vi "Generate_WF_Class_Dataset.vi"(8 "error in (no error)":errorcluster) -> (0 "error out":errorcluster, 3 "DataSets_All(In1D_Out1D)":T1={"Train"={"Inputs Ref."=variant(refnum<data-value> refnum), "Outputs Ref."=refnum, "Dims_In"=0, "Dataset_Size"=0, "Dims_Out"=0, "Labels"=[], "File Paths"=[]}, "Validation"={"Inputs Ref."=variant(refnum<data-value> refnum), "Outputs Ref."=refnum, "Dims_In"=0, "Dataset_Size"=0, "Dims_Out"=0, "Labels"=[], "File Paths"=[]}, "Test"={"Inputs Ref."=variant(refnum<data-value> refnum), "Outputs Ref."=refnum, "Dims_In"=0, "Dataset_Size"=0, "Dims_Out"=0, "Labels"=[], "File Paths"=[]}})   [LabVIEW 2020]
uses:
  <vilib>/Ngene/Deep Learning Toolkit/Toolkit/NN_Data/API/DataSet/DataSet_Types/NN_DataSets_All(In1D_Out1D).ctl
  <vilib>/Ngene/Deep Learning Toolkit/Toolkit/NN_Data/API/DataSet/DataSet_Types/NN_DataSet(In1D_Out1D).ctl
  <vilib>/Ngene/Deep Learning Toolkit/Toolkit/NN_Data/Controls/DataRef_Types/2D/NN_Data_ref(2D_SGL).ctl
  <vilib>/Ngene/Deep Learning Toolkit/Toolkit/Deep_Learning_Toolkit_by_Ngene.lvlib
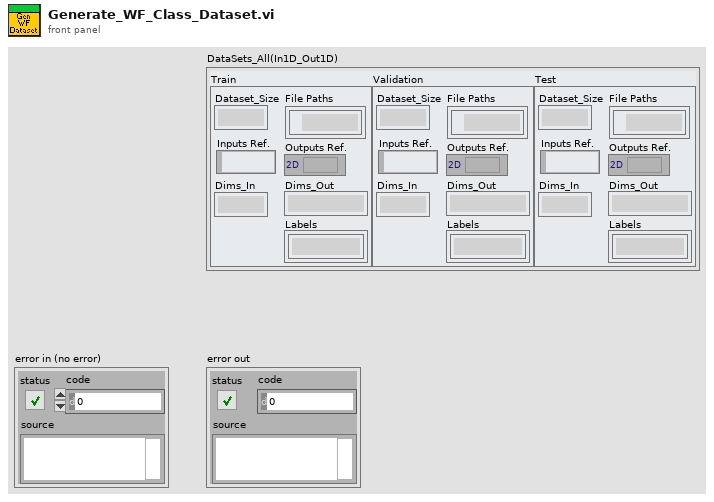
[diagram p1: front panel]
types:
  T1 = typedef "Deep_Learning_Toolkit_by_Ngene.lvlib/NN_DataSets_All(In1D_Out1D).ctl" = cluster{"Train":T2, "Validation":T2, "Test":T2}
  T2 = typedef "Deep_Learning_Toolkit_by_Ngene.lvlib/NN_DataSet(In1D_Out1D).ctl" = cluster{"Inputs Ref.":variant, "Outputs Ref.":T3, "Dims_In":i32, "Dataset_Size":i32, "Dims_Out":i32, "Labels":string[], "File Paths":path[]}
  T3 = typedef "Deep_Learning_Toolkit_by_Ngene.lvlib/NN_Data_ref(2D_SGL).ctl" = refnum<data-value>
  T4 = enum16{"Sine Wave", "Triangle Wave", "Square Wave", "Sawtooth Wave", "Noise"}[]
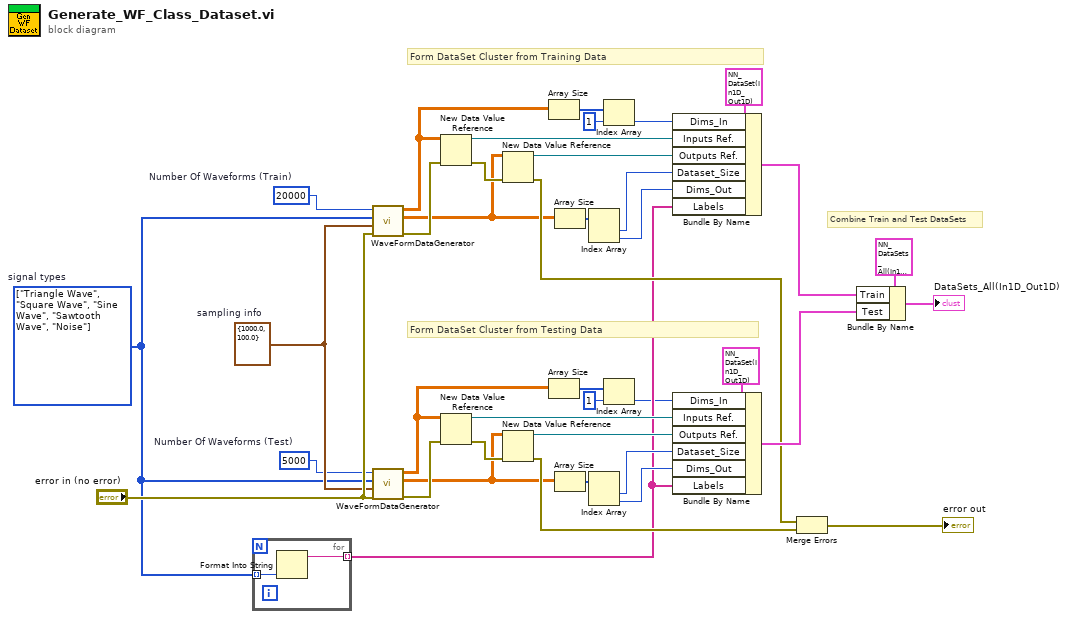
[diagram p0: block diagram]
diagram:
  w31 = 5000  # Number Of Waveforms (Test)
  w37 = cluster{"Fs":dbl, "#s":dbl} {"Fs"=1000.0, "#s"=100.0}  # sampling info
  w12 = 20000  # Number Of Waveforms (Train)
  w5 = T4 [enum."Triangle Wave", enum."Square Wave", enum."Sine Wave", enum."Sawtooth Wave", enum."Noise"] items=["Sine Wave", "Triangle Wave", "Square Wave", "Sawtooth Wave", "Noise"]  # signal types
  # "Combine Train and Test DataSets"
  # "Form DataSet Cluster from Testing Data"
  # "Form DataSet Cluster from Training Data"
  n1 = for {
    tunnel: w5 -> [w41] mode=indexing
    tunnel: [w40] -> w4 mode=indexing
    n2 = Format Into String(w41) -> (resulting string=w40:string)  [unwired: 3 in, 1 out]
  }
  n3 = call "WaveFormDataGenerator.vi"("error in"="error in (no error)", "sampling info"=w37, "Signal Types/Classes"=w5, "Number of Waveforms per Signal Type"=w12) -> ("error out"=w11:errorcluster, "One-Hot Encoded Labels"=w3:sgl[][], "Generated Waveform"=w15:sgl[][])  [unwired: 5 in]
  n4 = call "WaveFormDataGenerator.vi"("error in"="error in (no error)", "sampling info"=w37, "Signal Types/Classes"=w5, "Number of Waveforms per Signal Type"=w31) -> ("error out"=w32:errorcluster, "One-Hot Encoded Labels"=w25:sgl[][], "Generated Waveform"=w28:sgl[][])  [unwired: 5 in]
  n5 = New Data Value Reference(data value=w15, error in=w11) -> (data value reference=w14:refnum<data-value>, error out=w6:errorcluster)
  n6 = New Data Value Reference(data value=w28, error in=w32) -> (data value reference=w29:refnum<data-value>, error out=w35:errorcluster)
  n7 = New Data Value Reference(data value=w3, error in=w6) -> (data value reference=w13:refnum<data-value>, error out=w10:errorcluster)
  n8 = New Data Value Reference(data value=w25, error in=w35) -> (data value reference=w30:refnum<data-value>, error out=w33:errorcluster)
  n9 = Array Size(array=w15) -> (size(s)=w16:i32[])
  n10 = Array Size(array=w28) -> (size(s)=w27:i32[])
  n11 = Array Size(array=w3) -> (size(s)=w17:i32[])
  n12 = Array Size(array=w25) -> (size(s)=w26:i32[])
  n13 = Index Array(array=w17) -> (element #1=w20:i32, element #2=w18:i32)  [unwired: 2 in]
  n14 = Index Array(array=w26) -> (element #1=w22:i32, element #2=w24:i32)  [unwired: 2 in]
  n15 = Index Array(array=w16, index=1) -> (element=w1:i32)
  n16 = Index Array(array=w27, index=1) -> (element=w2:i32)
  n17 = Bundle By Name(cluster=T2 {"Inputs Ref."=variant(refnum<data-value> refnum), "Outputs Ref."=refnum, "Dims_In"=0, "Dataset_Size"=0, "Dims_Out"=0, "Labels"=[], "File Paths"=[]} ("Dataset(In1D_Out1D)"), "Dims_In"=w1, "Inputs Ref."=w14, "Outputs Ref."=w13, "Dataset_Size"=w20, "Dims_Out"=w18, "Labels"=w4) -> (w9:T2)
  n18 = Bundle By Name(cluster=T2 {"Inputs Ref."=variant(refnum<data-value> refnum), "Outputs Ref."=refnum, "Dims_In"=0, "Dataset_Size"=0, "Dims_Out"=0, "Labels"=[], "File Paths"=[]} ("Dataset(In1D_Out1D)"), "Dims_In"=w2, "Inputs Ref."=w29, "Outputs Ref."=w30, "Dataset_Size"=w22, "Dims_Out"=w24, "Labels"=w4) -> (w36:T2)
  n19 = Merge Errors(w10, w33) -> (→"error out":errorcluster)
  n20 = Bundle By Name(cluster=T1 {"Train"={"Inputs Ref."=variant(refnum<data-value> refnum), "Outputs Ref."=refnum, "Dims_In"=0, "Dataset_Size"=0, "Dims_Out"=0, "Labels"=[], "File Paths"=[]}, "Validation"={"Inputs Ref."=variant(refnum<data-value> refnum), "Outputs Ref."=refnum, "Dims_In"=0, "Dataset_Size"=0, "Dims_Out"=0, "Labels"=[], "File Paths"=[]}, "Test"={"Inputs Ref."=variant(refnum<data-value> refnum), "Outputs Ref."=refnum, "Dims_In"=0, "Dataset_Size"=0, "Dims_Out"=0, "Labels"=[], "File Paths"=[]}} ("DataSets_All(In1D_Out1D)"), "Train"=w9, "Test"=w36) -> (→"DataSets_All(In1D_Out1D)":T1)
